vi "Set A0 Chan Gain Property Node (24bit).vi"(8 "error in (no error)":errorcluster, 11 "AO Tasks":T1[](array[typedef])) -> (0 "error out":errorcluster)   [LabVIEW 2015]
uses:
  PXI Globals.vi
  <resource>/objmgr/daqmx.rc
  Type Defs/Task Struct.ctl
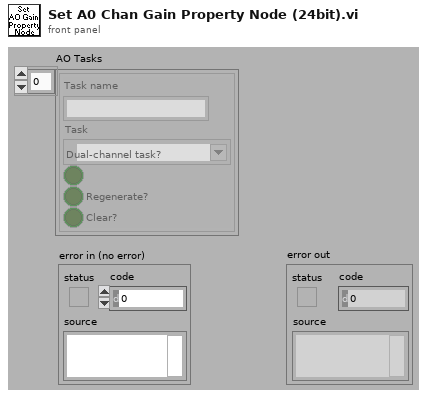
[diagram p1: front panel]
types:
  T1 = typedef "Task Struct.ctl" = cluster{"Task name":string, "Task":refnum<k21>, "Dual-channel task?":bool, "Regenerate?":bool, "Clear?":bool}
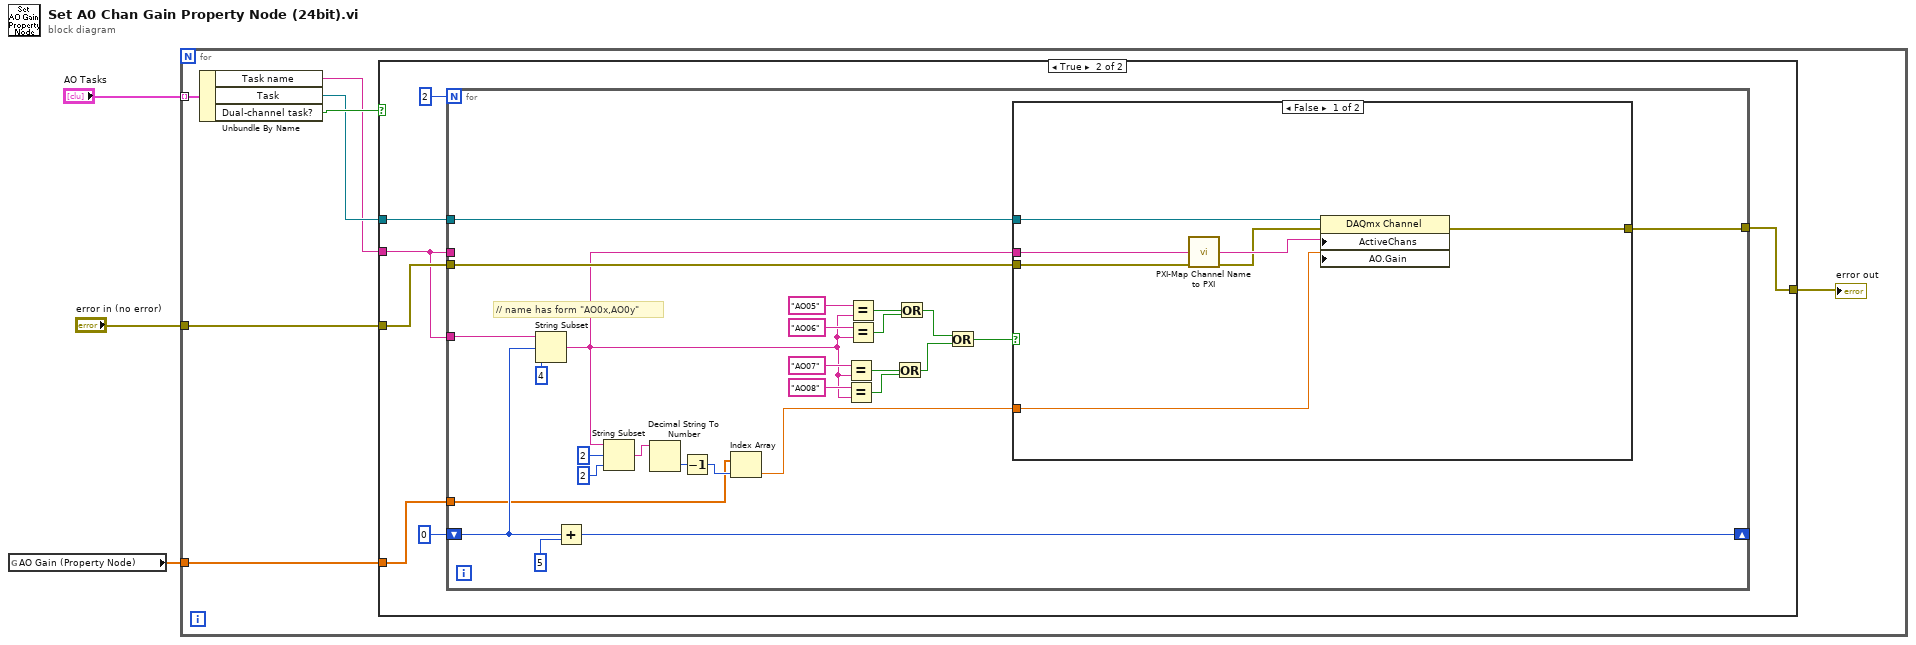
[diagram p0: block diagram]
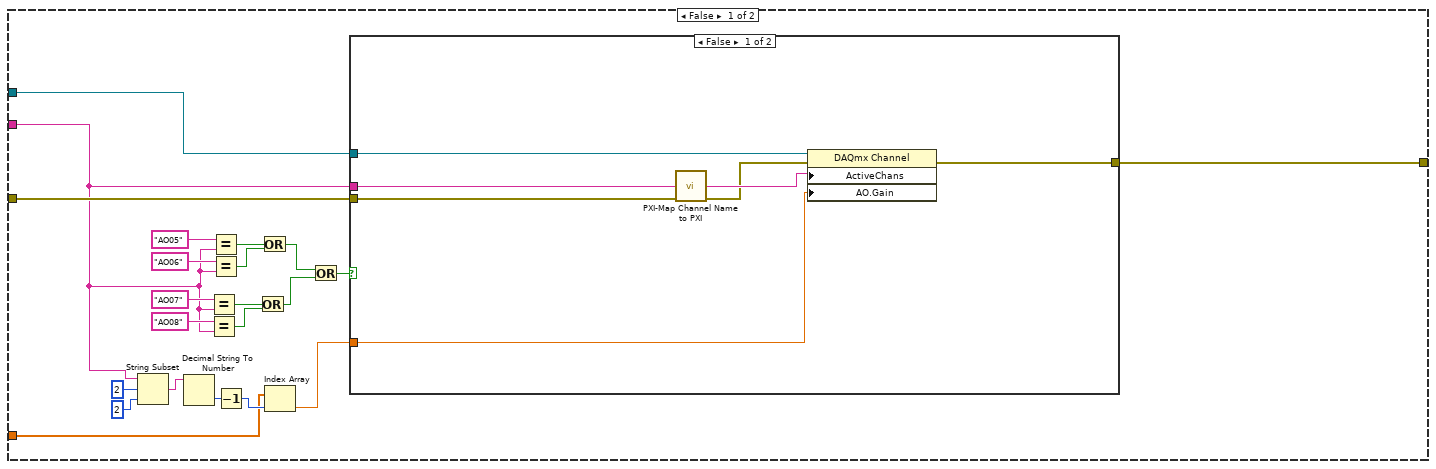
[diagram p2: hidden frame]
diagram:
  n1 = global read "PXI Globals.vi" "AO Gain (Property Node)"() -> (w3:dbl[])
  n2 = for {
    tunnel: "AO Tasks" -> [w10] mode=indexing
    tunnel: w3 -> [w6]
    tunnel: "error in (no error)" -> [w5]
    n3 = Unbundle By Name(w10) -> ("Task name"=w4:string, "Task"=w7:refnum<k21>, "Dual-channel task?"=w9:bool)
    n4 = case shown="True" w9 {
      tunnel: w4 -> [w11 w41]
      tunnel: [w15 w42] -> w8
      tunnel: w7 -> [w14 w43]
      tunnel: w6 -> [w13 w45]
      tunnel: w5 -> [w12 w44]
      frame False {
        n5 = String Subset(string=w11, offset (0)=2 ("length (rest)"), length (rest)=2) -> (substring=w21:string)
        n6 = Decimal String To Number(string=w21) -> (number=w19:i32)  [unwired: 2 in, 1 out]
        n7 = Equal?(x="AO07" ("Local Terminal Name"), y=w11) -> (x = y?=w27:bool)
        n8 = Equal?(x="AO08" ("Local Terminal Name"), y=w11) -> (x = y?=w28:bool)
        n9 = Equal?(x="AO05" ("Local Terminal Name"), y=w11) -> (x = y?=w31:bool)
        n10 = Equal?(x="AO06" ("Local Terminal Name"), y=w11) -> (x = y?=w32:bool)
        n11 = Decrement(x=w19) -> (x-1=w18:i32)
        n12 = Or(x=w27, y=w28) -> (x .or. y?=w24:bool)
        n13 = Or(x=w31, y=w32) -> (x .or. y?=w23:bool)
        n14 = Index Array(array=w13, index=w18) -> (element=w17:dbl)
        n15 = Or(x=w23, y=w24) -> (x .or. y?=w22:bool)
        n16 = case shown="False" w22 {
          tunnel: w14 -> [w35 _]
          tunnel: w11 -> [w34 _]
          tunnel: [w37 w40] -> w15
          tunnel: w17 -> [w36 _]
          tunnel: w12 -> [w33 w40]
          frame False {
            n17 = call "PXI-Map Channel Name to PXI.vi"("Channel"=w34, "error in (no error)"=w33) -> ("Physical Channel"=w39:tag, "error out"=w38:errorcluster)  [unwired: 12 in]
            n18 = property class="DAQmx Channel"(reference=w35, error in=w38, "ActiveChans"=w39, "AO.Gain"=w36) -> (error out=w37:errorcluster)  [unwired: 1 out]
          }
          frame True {
          }
        }
      }
      frame True {
        n19 = for {
          N: 2 -> [_]
          tunnel: w41 -> [w74]
          shift-right: [w72] -> _
          shift-left: 0 -> [w70]
          tunnel: w45 -> [w52]
          tunnel: w44 -> [w51]
          tunnel: w43 -> [w50]
          tunnel: [w49] -> w42
          tunnel: w41 -> [_]
          # "// name has form \"AO0x,AO0y\""
          n20 = String Subset(string=w74, offset (0)=w70, length (rest)=4 ("length (rest)")) -> (substring=w48:string)
          n21 = Add(x=w70, y=5) -> (x+y=w72:i32)
          n22 = String Subset(string=w48, offset (0)=2 ("length (rest)"), length (rest)=2) -> (substring=w58:string)
          n23 = Decimal String To Number(string=w58) -> (number=w56:i32)  [unwired: 2 in, 1 out]
          n24 = Decrement(x=w56) -> (x-1=w55:i32)
          n25 = Index Array(array=w52, index=w55) -> (element=w54:dbl)
          n26 = Equal?(x="AO07" ("Local Terminal Name"), y=w48) -> (x = y?=w64:bool)
          n27 = Equal?(x="AO08" ("Local Terminal Name"), y=w48) -> (x = y?=w65:bool)
          n28 = Equal?(x="AO05" ("Local Terminal Name"), y=w48) -> (x = y?=w68:bool)
          n29 = Equal?(x="AO06" ("Local Terminal Name"), y=w48) -> (x = y?=w69:bool)
          n30 = Or(x=w64, y=w65) -> (x .or. y?=w61:bool)
          n31 = Or(x=w68, y=w69) -> (x .or. y?=w60:bool)
          n32 = Or(x=w60, y=w61) -> (x .or. y?=w59:bool)
          n33 = case shown="False" w59 {
            tunnel: w50 -> [w77 _]
            tunnel: [w79 w82] -> w49
            tunnel: w54 -> [w78 _]
            tunnel: w48 -> [w76 _]
            tunnel: w51 -> [w75 w82]
            frame False {
              n34 = call "PXI-Map Channel Name to PXI.vi"("Channel"=w76, "error in (no error)"=w75) -> ("Physical Channel"=w81:tag, "error out"=w80:errorcluster)  [unwired: 12 in]
              n35 = property class="DAQmx Channel"(reference=w77, error in=w80, "ActiveChans"=w81, "AO.Gain"=w78) -> (error out=w79:errorcluster)  [unwired: 1 out]
            }
            frame True {
            }
          }
        }
      }
    }
    "error out" <- w8
  }
